vi "排序函数.vi"() -> ()   [LabVIEW 2012]
panel:
  out "降序排列数组":dbl[](array[numeric])
  out "升序排列数组":dbl[](array[numeric])
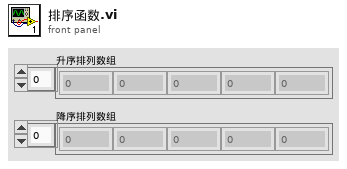
[diagram p1: front panel]
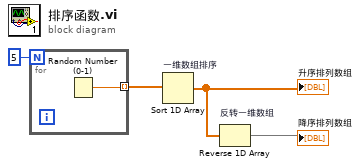
[diagram p0: block diagram]
diagram:
  n1 = for {
    N: 5 -> [_]
    tunnel: [w5] -> w3 mode=indexing
    n2 = Random Number (0-1)() -> (number: 0 to 1=w5:dbl)
  }
  n3 = Sort 1D Array "一维数组排序"(array=w3) -> (sorted array=w2:dbl[])
  "升序排列数组" <- w2
  n4 = Reverse 1D Array "反转一维数组"(array=w2) -> (reversed array=→"降序排列数组":dbl[])
